vi "DO Camera.vi"() -> ()   [LabVIEW 2020]
uses:
  <vilib>/DAQmx/create/channels.llb/DAQmx Create Channel (CO-Pulse Generation-Frequency).vi
  <vilib>/DAQmx/configure/timing.llb/DAQmx Timing (Sample Clock).vi
  <vilib>/DAQmx/write.llb/DAQmx Write (Counter 1D Frequency 1Chan NSamp).vi
panel:
  in  "Boolean":bool
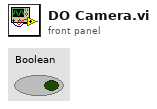
[diagram p1: front panel]
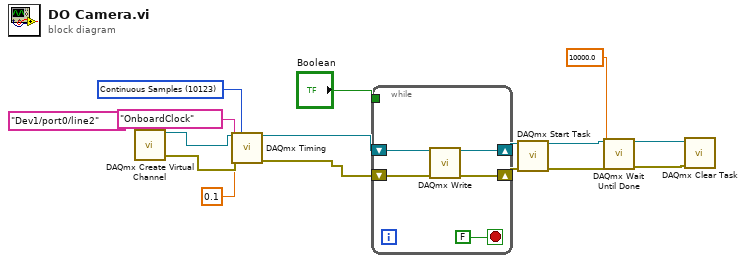
[diagram p0: block diagram]
diagram:
  w16 = 10123 items=["Finite Samples"=10178, "Continuous Samples"=10123, "Hardware Timed Single Point"=12522] ("sample mode")
  n1 = call-poly <vilib>:"DAQmx Create Virtual Channel.vi"("counter"=tag "Dev1/port0/line2" ("lines")) -> ("task out"=w15:refnum<k21>, "error out"=w14:errorcluster)  [unwired: 13 in]
  n2 = call-poly <vilib>:"DAQmx Timing.vi"("task/channels in"=w15, "sample mode"=w16, "rate"=0.1, "source"=tag "OnboardClock", "error in"=w14) -> ("task out"=w3:refnum<k21>, "error out"=w4:errorcluster)  [unwired: 9 in]
  n3 = while {
    shift-right: [w19] -> w9
    shift-left: w4 -> [w21]
    shift-right: [w20] -> w12
    shift-left: w3 -> [w17]
    tunnel: "Boolean" -> [_]
    stop <- FALSE stop-if-true
    n4 = call-poly <vilib>:"DAQmx Write.vi"("task/channels in"=w17, "error in"=w21) -> ("task out"=w20:refnum<k21>, "error out"=w19:errorcluster)  [unwired: 11 in, 1 out]
  }
  n5 = call <vilib>:"DAQmx Start Task.vi"("task/channels in"=w12, "error in"=w9) -> ("task out"=w11:refnum<k21>, "error out"=w8:errorcluster)  [unwired: 12 in]
  n6 = call <vilib>:"DAQmx Wait Until Done.vi"("task/channels in"=w11, "timeout (sec)"=10000.0, "error in"=w8) -> ("task out"=w10:refnum<k21>, "error out"=w7:errorcluster)  [unwired: 11 in]
  n7 = call <vilib>:"DAQmx Clear Task.vi"("task in"=w10, "error in"=w7) -> ()  [unwired: 13 in, 1 out]
